vi "Read MultipartData.vi"(8 "error in (no error)":errorcluster, 11 "httpRequest in":refnum<class "httpRequest.lvclass">) -> (0 "error out":errorcluster, 2 "Multipart Post data":T1[](array[typedef]), 3 "httpRequest out":refnum<class "httpRequest.lvclass">)   [LabVIEW 2020, in "httpClient.lvlib" / "httpRequest.lvclass"]
uses:
  httpRequest.lvclass
  Multipart data -- cluster.ctl
  httpRequest.lvclass/httpRequest.ctl
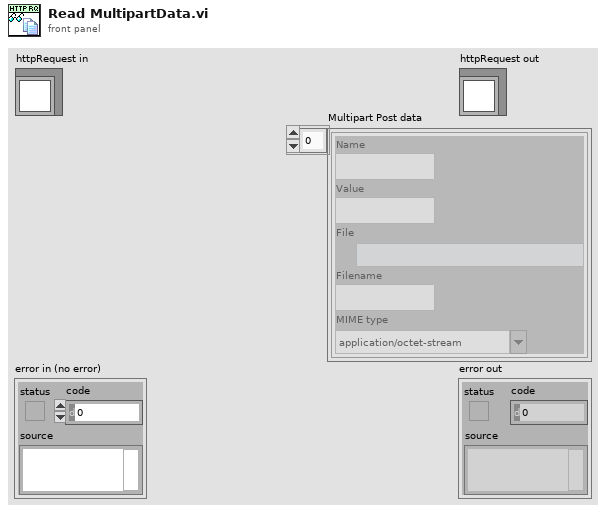
[diagram p1: front panel]
types:
  T1 = typedef "httpClient.lvlib/httpRequest.lvclass/Multipart data -- cluster.ctl" = cluster{"Name":string, "Value":string, "File":path, "Filename":string, "MIME type":string}
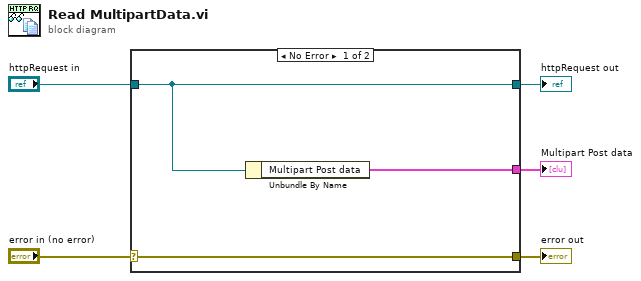
[diagram p0: block diagram]
diagram:
  n1 = case shown="No Error" "error in (no error)" {
    selector: "error in (no error)" -> [w8 w9]
    tunnel: [w8 w9] -> w4
    tunnel: [w7 w10] -> w2
    tunnel: "httpRequest in" -> [w7 w10]
    tunnel: [w6 _] -> w1
    frame No Error {
      n2 = Unbundle By Name(w7) -> ("Multipart Post data"=w6:T1[])
    }
    frame Error {
    }
  }
  "error out" <- w4
  "httpRequest out" <- w2
  "Multipart Post data" <- w1
